vi "Build Message Data.vi"(7 "Virtual Memory Unit in":refnum<class "Virtual Memory Unit.lvclass">, 8 "error in (no error)":errorcluster, 10 "Starting Address":u16 format="%04x", 11 "Message in":refnum<class "Message.lvclass">) -> (0 "error out":errorcluster, 2 "Next Available Address":u16 format="%04x", 3 "Message out":refnum<class "Message.lvclass">, 5 "Virtual Memory Unit out":refnum<class "Virtual Memory Unit.lvclass">)   [LabVIEW 2020, in "BCI-1553 API.lvlib" / "Message.lvclass"]
doc: "Initializes the data used by this message command. This can be for either receive or transmit."
uses:
  Message.lvclass
  Dependencies/Virtual Memory Unit/Virtual Memory Unit.lvclass
  Message.lvclass/Message.ctl
  BCI-1553 API.lvlib
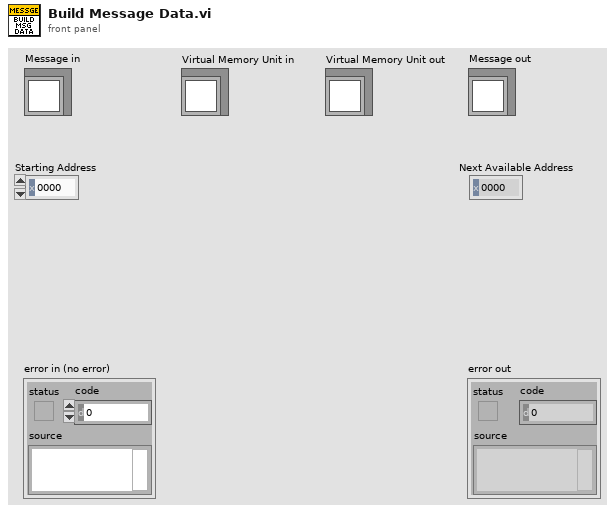
[diagram p1: front panel]
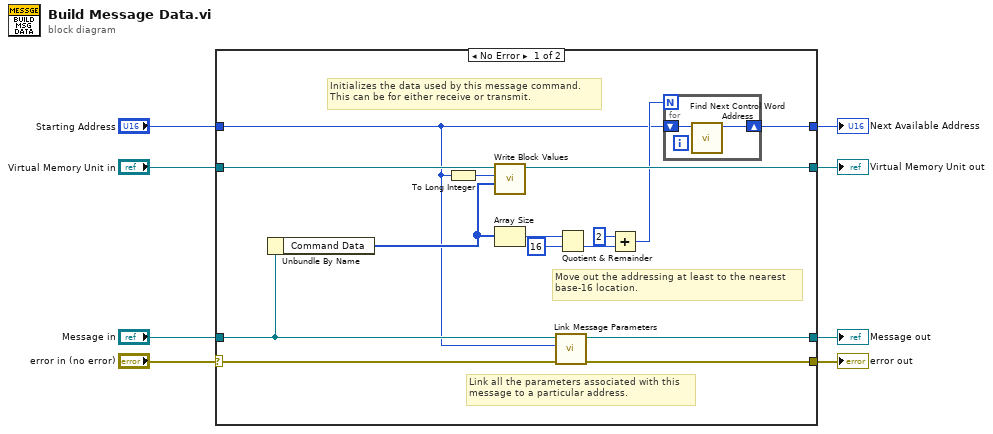
[diagram p0: block diagram]
diagram:
  n1 = case shown="No Error" "error in (no error)" {
    selector: "error in (no error)" -> [w15 w29]
    tunnel: [w14 w29] -> w7
    tunnel: [w12 w28] -> w5
    tunnel: "Message in" -> [w13 w28]
    tunnel: "Virtual Memory Unit in" -> [w22 w26]
    tunnel: "Starting Address" -> [w9 w27]
    tunnel: [w21 w26] -> w2
    tunnel: [w23 w27] -> w1
    frame No Error {
      # "Link all the parameters associated with this\nmessage to a particular address."
      # "Move out the addressing at least to the nearest\nbase-16 location."
      # "Initializes the data used by this message command.\nThis can be for either receive or transmit."
      n2 = Unbundle By Name(w13) -> ("Command Data"=w10:u16[])
      n3 = To Long Integer(number=w9) -> (32bit integer=w20:i32)
      n4 = call "Write Block Values.vi"("Write Block"=w10, "Start Index"=w20, "Virtual Memory Unit in"=w22) -> ("Virtual Memory Unit out"=w21:refnum<class "Virtual Memory Unit.lvclass">)  [unwired: 7 in, 1 out]
      n5 = Array Size(array=w10) -> (size(s)=w19:i32)
      n6 = call-dynamic "Link Message Parameters.vi"("error in (no error)"=w15, "Starting Address"=w9, "Message in"=w13) -> ("error out"=w14:errorcluster, "Message out"=w12:refnum<class "Message.lvclass">)  [unwired: 7 in]
      n7 = Quotient & Remainder(x=w19, y=16) -> (floor(x/y)=w17:i32)  [unwired: 1 out]
      n8 = Add(x=2, y=w17) -> (x+y=w16:i32)
      n9 = for {
        N: w16 -> [_]
        shift-right: [w25] -> w23
        shift-left: w9 -> [w24]
        n10 = call "Find Next Control Word Address.vi"("Starting Address"=w24) -> ("0xHHHX Address"=w25:u16)  [unwired: 10 in]
      }
    }
    frame Error {
    }
  }
  "error out" <- w7
  "Message out" <- w5
  "Virtual Memory Unit out" <- w2
  "Next Available Address" <- w1
